vi "Delete PID Parameter Row.vi"(8 "error in (no error)":errorcluster, 10 "Coords":T1, 11 "MulticolumnListbox in":refnum<vi>) -> (0 "error out":errorcluster)   [LabVIEW 2019, in "Control Addon Shared.lvlib"]
uses:
  Control Addon Shared.lvlib
  <vilib>/Utility/miscctls.llb/LVPoint32TypeDef.ctl
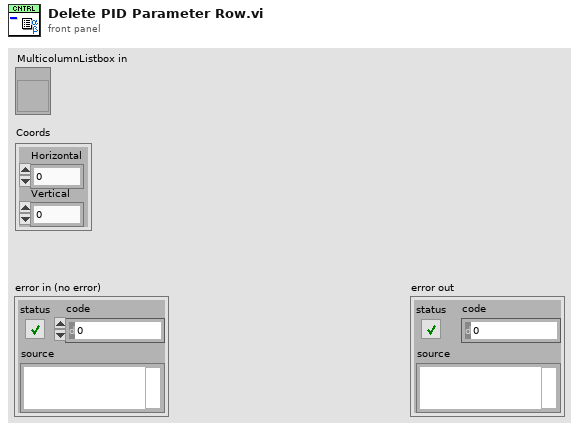
[diagram p1: front panel]
types:
  T1 = typedef "LVPoint32TypeDef.ctl" = cluster{"Horizontal":i32, "Vertical":i32}
  T2 = typedef "LVRowAndColumnTypeDef.ctl" = cluster{"Row":i32, "Column":i32}
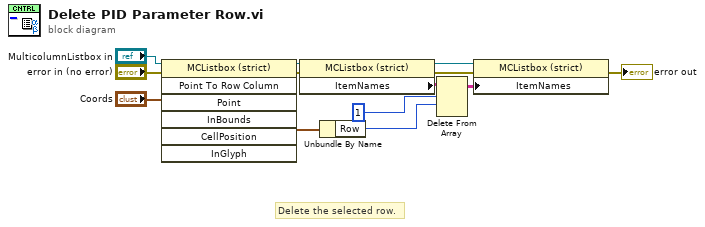
[diagram p0: block diagram]
diagram:
  # "Delete the selected row."
  n1 = invoke class="MCListbox (strict)" method="Point To Row Column"(reference="MulticolumnListbox in", error in="error in (no error)", "Point"="Coords") -> (reference out=w6:refnum<vi>, error out=w5:errorcluster, "CellPosition"=w10:T2)  [unwired: 4 in, 4 out]
  n2 = property class="MCListbox (strict)"(reference=w6, error in=w5) -> (reference out=w4:refnum<vi>, error out=w3:errorcluster, "ItemNames"=w7:string[][])
  n3 = Unbundle By Name(w10) -> ("Row"=w11:i32)
  n4 = Delete From Array(array=w7, length=1, index (row)=w11) -> (array with subset deleted=w8:string[][])  [unwired: 1 in, 1 out]
  n5 = property class="MCListbox (strict)"(reference=w4, error in=w3, "ItemNames"=w8) -> (error out=→"error out":errorcluster)  [unwired: 1 out]
